vi "demoautodrive.vi"() -> ()   [LabVIEW 2012, in "Demo.lvrbt"]
uses:
  Demo.lvrbt
  <vilib>/NXT/Dual Mode Library/Waits/Wait_Num(msec).vi
  <vilib>/NXT/LegoClasses/BrickReference/BrickReference.lvclass
  <vilib>/NXT/Subs/LVHSConnector.ctl
  <vilib>/NXT/NXTIO Xnodes/NXTIOXNode/NXTIO.xnode
  <vilib>/NXT/NXTIO Xnodes/AddressXNode/NXTIOAddress.xnode
  <vilib>/NXT/Hardware/Plugins/Tetrix DC Motor/TetrixDCMotorAddress.ctl
  <vilib>/NXT/NXTIO Xnodes/NXTIONodeSubVIs/TETRIX IO Move DC Motors.vi
  <vilib>/NXT/NXTIO Xnodes/NXTIONodeSubVIs/TETRIX IO Stop DC Motors.vi
panel:
  out "Enabled":bool
  out "iter":i32
  out "NXT":T1
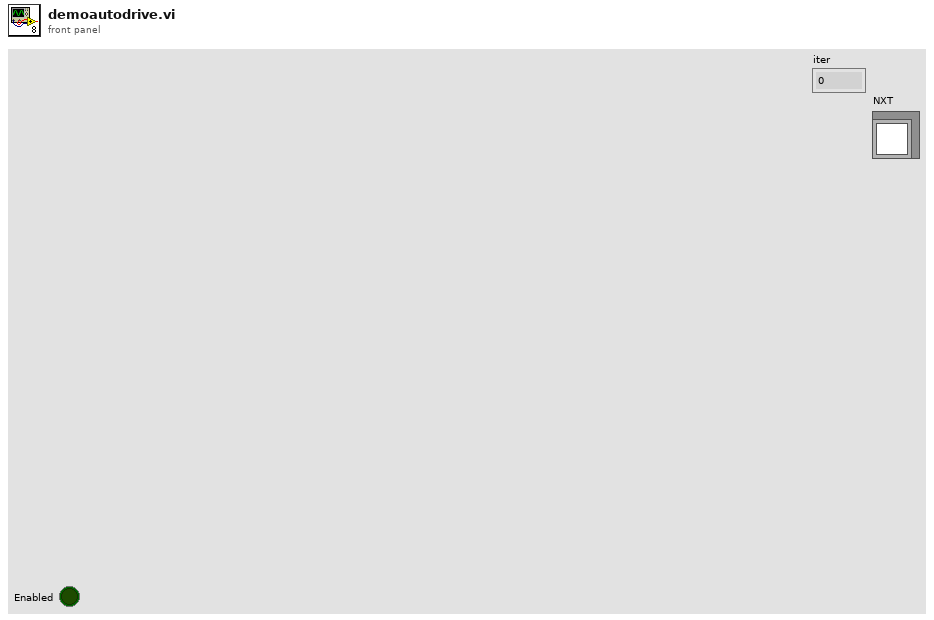
[diagram p1: front panel]
types:
  T1 = typedef "LVHSConnector.ctl" = refnum<class "BrickReference.lvclass">
  T2 = typedef "TetrixDCMotorAddress.ctl" = i16
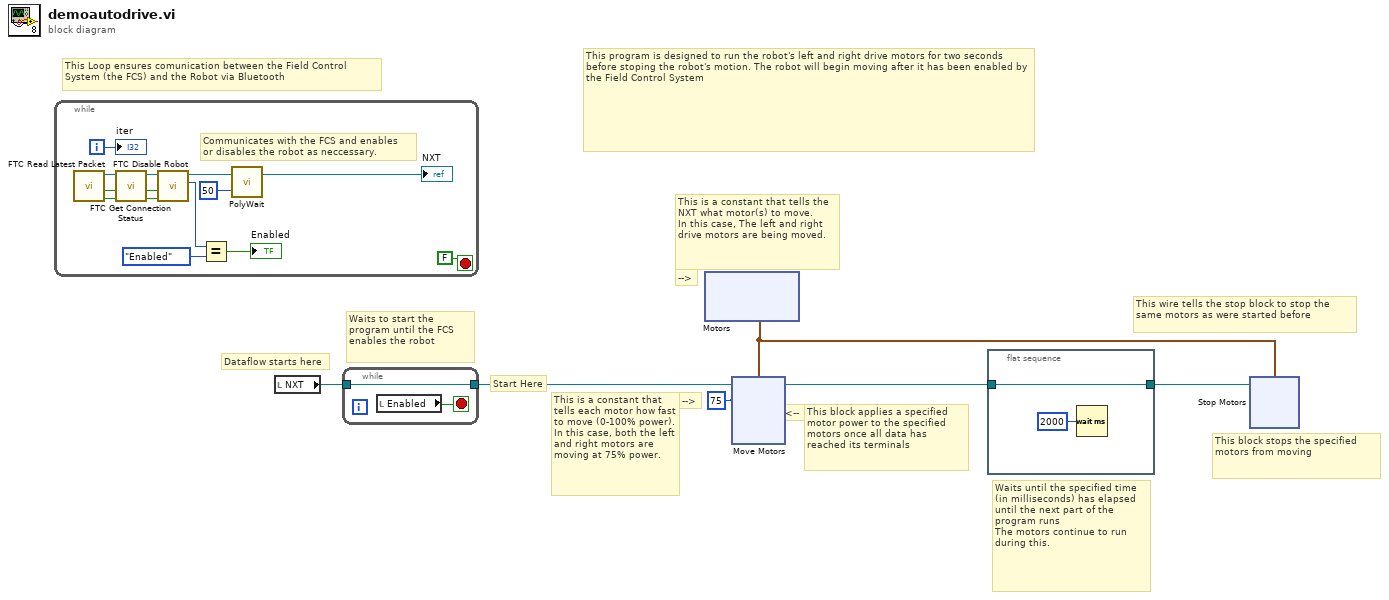
[diagram p0: block diagram]
diagram:
  w4 = i8 75 ("Power/Speed 1")
  # "This program is designed to run the robot's left and right drive motors for two seconds before stoping the robot's motion. The robot will begin moving after it has been enabled by the Field Control System"
  # "This block stops the specified motors from moving"
  # "This wire tells the stop block to stop the same motors as were started before"
  # "Waits until the specified time (in milliseconds) has elapsed until the next part of the program runs\nThe motors continue to run during this."
  # "<--"
  # "This block applies a specified motor power to the specified motors once all data has reached its terminals"
  # "-->"
  # "-->"
  # "This is a constant that tells each motor how fast to move (0-100% power). In this case, both the left and right motors are moving at 75% power."
  # "Dataflow starts here"
  # "This is a constant that tells the NXT what motor(s) to move.\nIn this case, The left and right drive motors are being moved."
  # "Waits to start the program until the FCS enables the robot"
  # "This Loop ensures comunication between the Field Control System (the FCS) and the Robot via Bluetooth"
  # "Start Here"
  n1 = while {
    i -> [w8]
    stop <- FALSE stop-if-true
    # "Communicates with the FCS and enables \nor disables the robot as neccessary."
    n2 = call <vilib>:"FTC Read Latest Packet.vi"() -> ("Packet Received?"=w18:bool, "Stopped?"=w17:bool, "NXT"=w20:T1)  [unwired: 6 in, 3 out]
    n3 = call <vilib>:"FTC Get Connection Status.vi"("Packet Received?"=w18, "Stopped?"=w17, "NXT"=w20) -> ("Online?"=w10:bool, "Stopped?"=w11:bool, "NXT"=w19:T1)  [unwired: 5 in]
    n4 = call <vilib>:"FTC Disable Robot.vi"("Online?"=w10, "Stopped?"=w11, "NXT"=w19) -> ("Enabled?"=w14:enum16{"Disabled", "Enabled"}, "NXT"=w16:T1)  [unwired: 3 in]
    n5 = Equal?(x=w14, y=enum16{"Disabled", "Enabled"}."Enabled") -> (x = y?=→"Enabled":bool)
    n6 = call-poly <vilib>:"PolyWait.vi"("Time (100 msec)"=u32 50 ("Time (msec)"), "NXT"=w16) -> ("NXT"=→"NXT":T1)  [unwired: 2 in]
    "iter" <- w8
  }
  n7 = local read "NXT"() -> (w6:T1)
  n8 = while {
    tunnel: w6 -> [w21]
    tunnel: [w21] -> w5
    stop <- w22 stop-if-true
    n9 = local read "Enabled"() -> (w22:bool)
  }
  n10 = xnode "Motors"() -> ("Motor"=w1:cluster{"TetrixDCMotor":T2, "TetrixDCMotor":T2})
  n11 = xnode "Move Motors"("Power/Speed 2"=w4, "Power/Speed 1"=w4, "Motors"=w1, "NXT/EV3"=w5) -> ("NXT/EV3"=w3:T1)
  n12 = flat-sequence {
    tunnel: w3 -> [w24]
    tunnel: [w24] -> w2
    frame #0 {
      n13 = Wait (ms)(milliseconds to wait=u32 2000) -> ()  [unwired: 1 out]
    }
  }
  n14 = xnode "Stop Motors"("Motors"=w1, "NXT/EV3"=w2) -> ()  [unwired: 1 out]
